vi "tb_run_test_sequence.vi"() -> ()   [LabVIEW 2019]
doc: "This VI performs a sequence of measurements defined in the Test vector (ctl_test_vector_array type).\nThe array items are queued in a Producer-Consumer structure and the dequeued in the Consumer loop, performing a single measurement by the run_test_item VI.\nWhen each measurements were done, the results are written into a Log file using the write_to_logfile VI"
uses:
  ctl_results_array.ctl
  ctl_results_cluster.ctl
  ctl_pass_fail_led.ctl
  ctl_test_outputs_cluster.ctl
  ctl_test_item_cluster.ctl
  ctl_stimuli_cluster.ctl
  ctl_loads_enum.ctl
  ctl_pass_limits_cluster.ctl
  ctl_test_vector_array.ctl
panel:
  in  "DAQmx Device Name":tag="Dev1"
  in  "Log file":path
  out "Outputs":T1[](array[typedef])
  out "Test sequence results":T2 {"Time Stamp" format="%<%.3X>T"}
  in  "Test vector":path
  out "Total test count":i32
  out "Test processed":i32
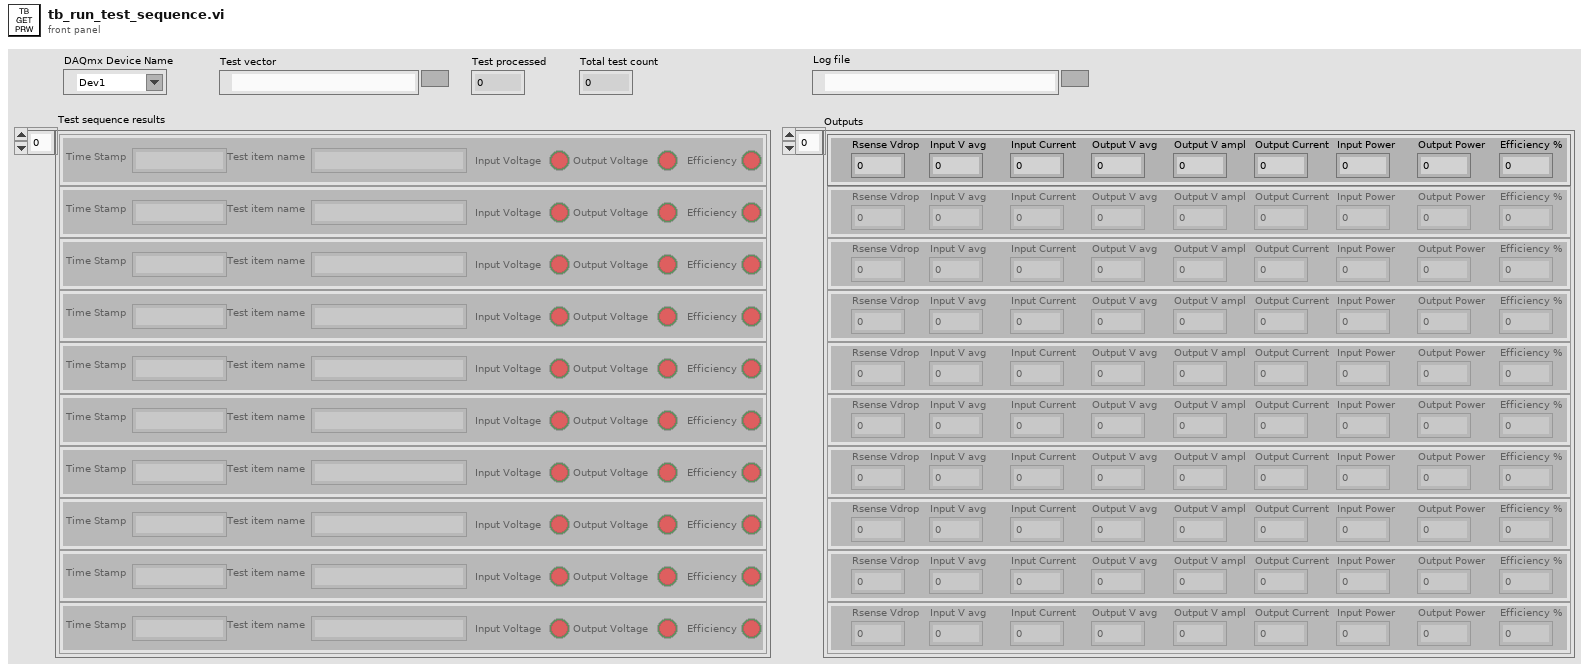
[diagram p1: front panel]
types:
  T1 = typedef "ctl_test_outputs_cluster.ctl" = cluster{"Output V avg":dbl, "Output V ampl":dbl, "Input Current":dbl, "Output Current":dbl, "Efficiency %":dbl, "Input V avg":dbl, "Input Power":dbl, "Output Power":dbl, "Rsense Vdrop":dbl}
  T2 = typedef "ctl_results_array.ctl" = T3[]
  T3 = typedef "ctl_results_cluster.ctl" = cluster{"Time Stamp":timestamp, "Test item name":string, "Input Voltage":T4, "Output Voltage":T4, "Efficiency":T4}
  T4 = typedef "ctl_pass_fail_led.ctl" = bool
  T5 = typedef "ctl_test_vector_array.ctl" = T6[]
  T6 = typedef "ctl_test_item_cluster.ctl" = cluster{"Stimuli":T7, "Pass limits":T9, "Test item name":string}
  T7 = typedef "ctl_stimuli_cluster.ctl" = cluster{"Load":T8, "Rsense Value":dbl}
  T8 = typedef "ctl_loads_enum.ctl" = enum16{"1.3 Ohm", "3.3 Ohm", "4.7 Ohm", "6.8 Ohm", "10 Ohm", "NO LOAD"}
  T9 = typedef "ctl_pass_limits_cluster.ctl" = cluster{"Output V avg":dbl, "Output V ampl max":dbl, "Efficiency min":dbl, "Input V min":dbl, "Output V avg range":dbl}
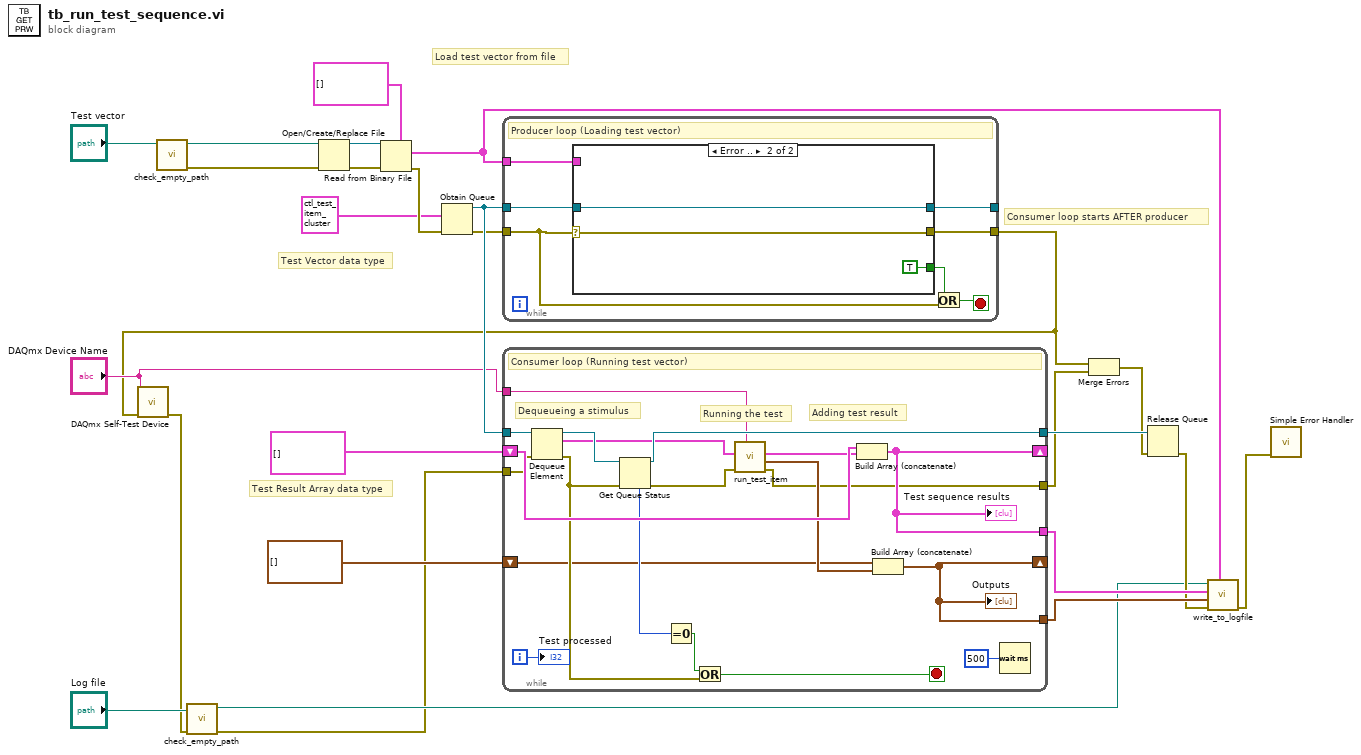
[diagram p0: block diagram]
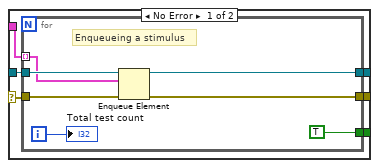
[diagram p2: hidden frame]
diagram:
  # "Consumer loop starts AFTER producer"
  # "Test Result Array data type"
  # "Test Vector data type"
  # "Load test vector from file"
  n1 = call "check_empty_path.vi"("Path to check"="Test vector") -> ("error out"=w6:errorcluster, "Path to check out"=w5:path)  [unwired: 9 in]
  n2 = Open/Create/Replace File(file path (use dialog)=w5, error in=w6) -> (refnum out=w25:refnum<file>, error out=w24:errorcluster)  [unwired: 4 in, 1 out]
  n3 = Read from Binary File(5:T5 [] ("Test vector"), 8:w24, 11:w25) -> (0:w19:errorcluster, 2:w10:T5)  [unwired: 3 in, 2 out]
  n4 = Obtain Queue(element data type=T6 {"Stimuli"={"Load"=enum."1.3 Ohm", "Rsense Value"=0.0}, "Pass limits"={"Output V avg"=0.0, "Output V ampl max"=0.0, "Efficiency min"=0.0, "Input V min"=0.0, "Output V avg range"=0.0}, "Test item name"=""} ("Test item"), error in (no error)=w19) -> (queue out=w26:refnum<queue>, error out=w23:errorcluster)  [unwired: 3 in, 1 out]
  n5 = while {
    tunnel: w26 -> [w32]
    tunnel: w10 -> [w33]
    tunnel: [w31] -> _
    tunnel: w23 -> [w27]
    tunnel: [w30] -> w8
    stop <- w29 stop-if-true
    # "Producer loop (Loading test vector)"
    n6 = case shown="Error .." w27 {
      selector: w27 -> [w34 w48]
      tunnel: w33 -> [w39 _]
      tunnel: w32 -> [w38 w49]
      tunnel: [w37 w49] -> w31
      tunnel: [w36 w48] -> w30
      tunnel: [w35 TRUE] -> w28
      frame No Error {
        n7 = for {
          tunnel: w39 -> [w45] mode=indexing
          tunnel: w38 -> [w46]
          tunnel: [w44] -> w37
          tunnel: w34 -> [w43]
          tunnel: [w42] -> w36
          tunnel: [TRUE] -> w35
          i -> [w40]
          # "Enqueueing a stimulus"
          n8 = Enqueue Element(queue=w46, element=w45, error in (no error)=w43) -> (queue out=w44:refnum<queue>, error out=w42:errorcluster)  [unwired: 1 in, 1 out]
          "Total test count" <- w40
        }
      }
      frame Error {
      }
    }
    n9 = Or(x=w28, y=w27) -> (x .or. y?=w29:bool)
  }
  n10 = call <vilib>:"DAQmx Self-Test Device.vi"("device in"="DAQmx Device Name", "error in"=w8) -> ("error out"=w2:errorcluster)  [unwired: 13 in]
  n11 = call "check_empty_path.vi"("error in"=w2, "Path to check"="Log file") -> ("error out"=w1:errorcluster, "Path to check out"=w3:path)  [unwired: 8 in]
  n12 = while {
    tunnel: w26 -> [w69]
    shift-right: [w54] -> _
    shift-left: T2 [] ("Test sequence results") -> [w67]
    tunnel: [w61] -> w22
    tunnel: [w50] -> w21
    tunnel: w1 -> [w59]
    shift-right: [w53] -> _
    shift-left: T1[] [] -> [w55]
    tunnel: [w54] -> w14
    tunnel: [w53] -> w13
    tunnel: "DAQmx Device Name" -> [w52]
    i -> [w68]
    stop <- w64 stop-if-true
    # "Adding test result"
    # "Running the test"
    # "Dequeueing a stimulus"
    # "Consumer loop (Running test vector)"
    n13 = Dequeue Element(queue=w69, error in (no error)=w59) -> (queue out=w63:refnum<queue>, element=w58:T6, error out=w60:errorcluster)  [unwired: 1 in, 1 out]
    n14 = Get Queue Status(queue=w63, error in (no error)=w60) -> (queue out=w61:refnum<queue>, error out=w51:errorcluster, # elements in queue=w62:i32)  [unwired: 1 in, 5 out]
    n15 = Equal To 0?(x=w62) -> (x = 0?=w65:bool)
    n16 = Or(x=w65, y=w60) -> (x .or. y?=w64:bool)
    n17 = call "run_test_item.vi"("DAQmx Device Name"=w52, "error in"=w51, "Test item"=w58) -> ("error out"=w50:errorcluster, "Test result"=w56:T1, "Cluster"=w57:T3)  [unwired: 6 in]
    n18 = Build Array (concatenate)(w67, w57) -> (w54:T2)
    "Test sequence results" <- w54
    n19 = Build Array (concatenate)(w55, w56) -> (w53:T1[])
    "Outputs" <- w53
    n20 = Wait (ms)(milliseconds to wait=u32 500) -> ()  [unwired: 1 out]
    "Test processed" <- w68
  }
  n21 = Merge Errors(w8, w21) -> (w20:errorcluster)
  n22 = Release Queue(queue=w22, error in (no error)=w20) -> (error out=w12:errorcluster)  [unwired: 1 in, 2 out]
  n23 = call "write_to_logfile.vi"("Test vector"=w10, "error in (no error)"=w12, "Array"=w13, "Test sequence results"=w14, "Log file"=w3) -> ("error out"=w11:errorcluster)  [unwired: 6 in]
  n24 = call <vilib>:"Simple Error Handler.vi"("error in (no error)"=w11) -> ()  [unwired: 4 in, 5 out]
